vi "Read Enabled Values.vi"(8 "error in (no error)":errorcluster, 11 "Output in":refnum<class "Output.lvclass">) -> (0 "error out":errorcluster, 1 "Data Values Native":dbl[](array[numeric]), 2 "Data Values Engineering":dbl[](array[numeric]), 3 "Output out":refnum<class "Output.lvclass">)   [LabVIEW 2018, in "Output.lvclass"]
uses:
  Output.lvclass
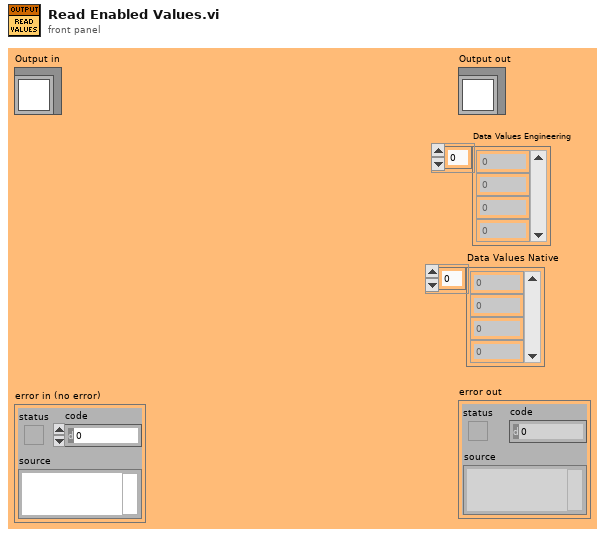
[diagram p1: front panel]
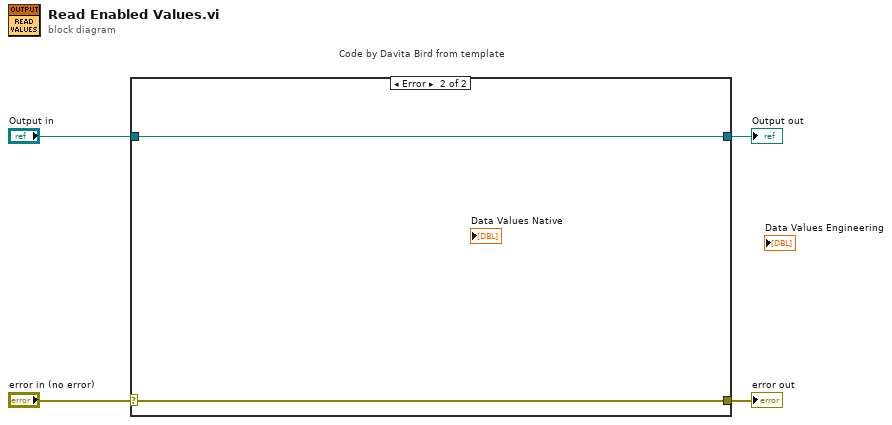
[diagram p0: block diagram]
diagram:
  n1 = case "Code by Davita Bird from template" shown="Error" "error in (no error)" {
    selector: "error in (no error)" -> [w5 w8]
    tunnel: [w5 w8] -> w3
    tunnel: [w6 w7] -> w1
    tunnel: "Output in" -> [w6 w7]
    frame No Error {
    }
    frame Error {
    }
  }
  "error out" <- w3
  "Output out" <- w1
